vi "TCP.IP Server for Ripple Detection - Experiment 6.vi"() -> ()   [LabVIEW 2021]
doc: "Demonstrates how to set up a basic TCP connection, send data to the specified port once a connection has been established, and terminate the connection once the data has been sent. This VI is designed to stop if the TCP connection is terminated. The data sent in this example is an array of random numbers."
panel:
  in  "Number of row to read \nat a time":i32=10000
  in  "File Path":path
  out "Iteration terminal":i32
  in  "Stop 2":bool
  in  "Client Closed":string="The client VI closed the connection."
  in  "Stop":bool
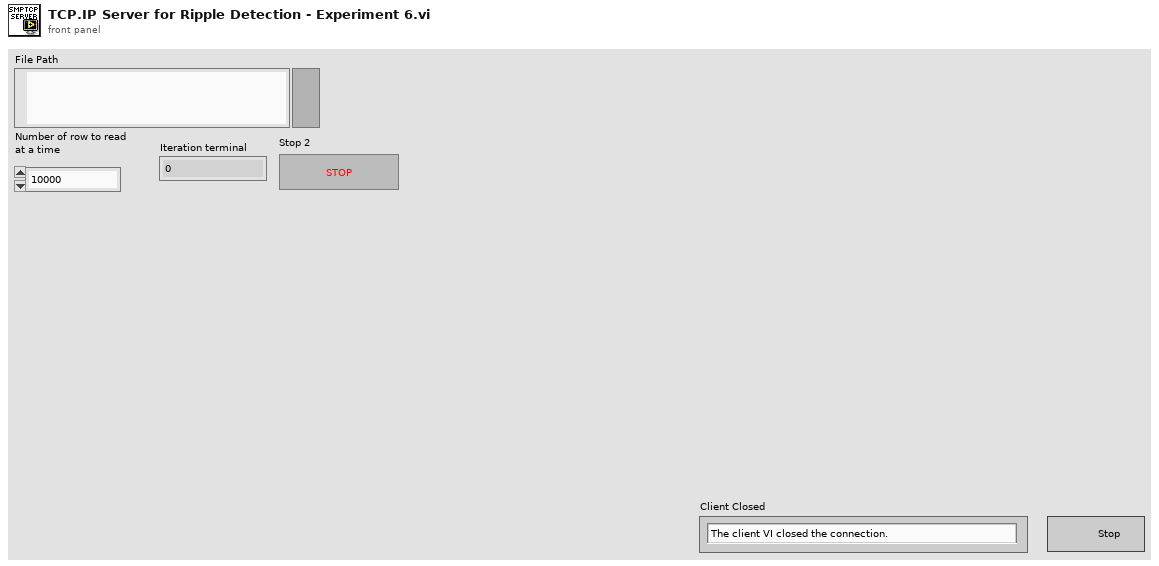
[diagram p1: front panel]
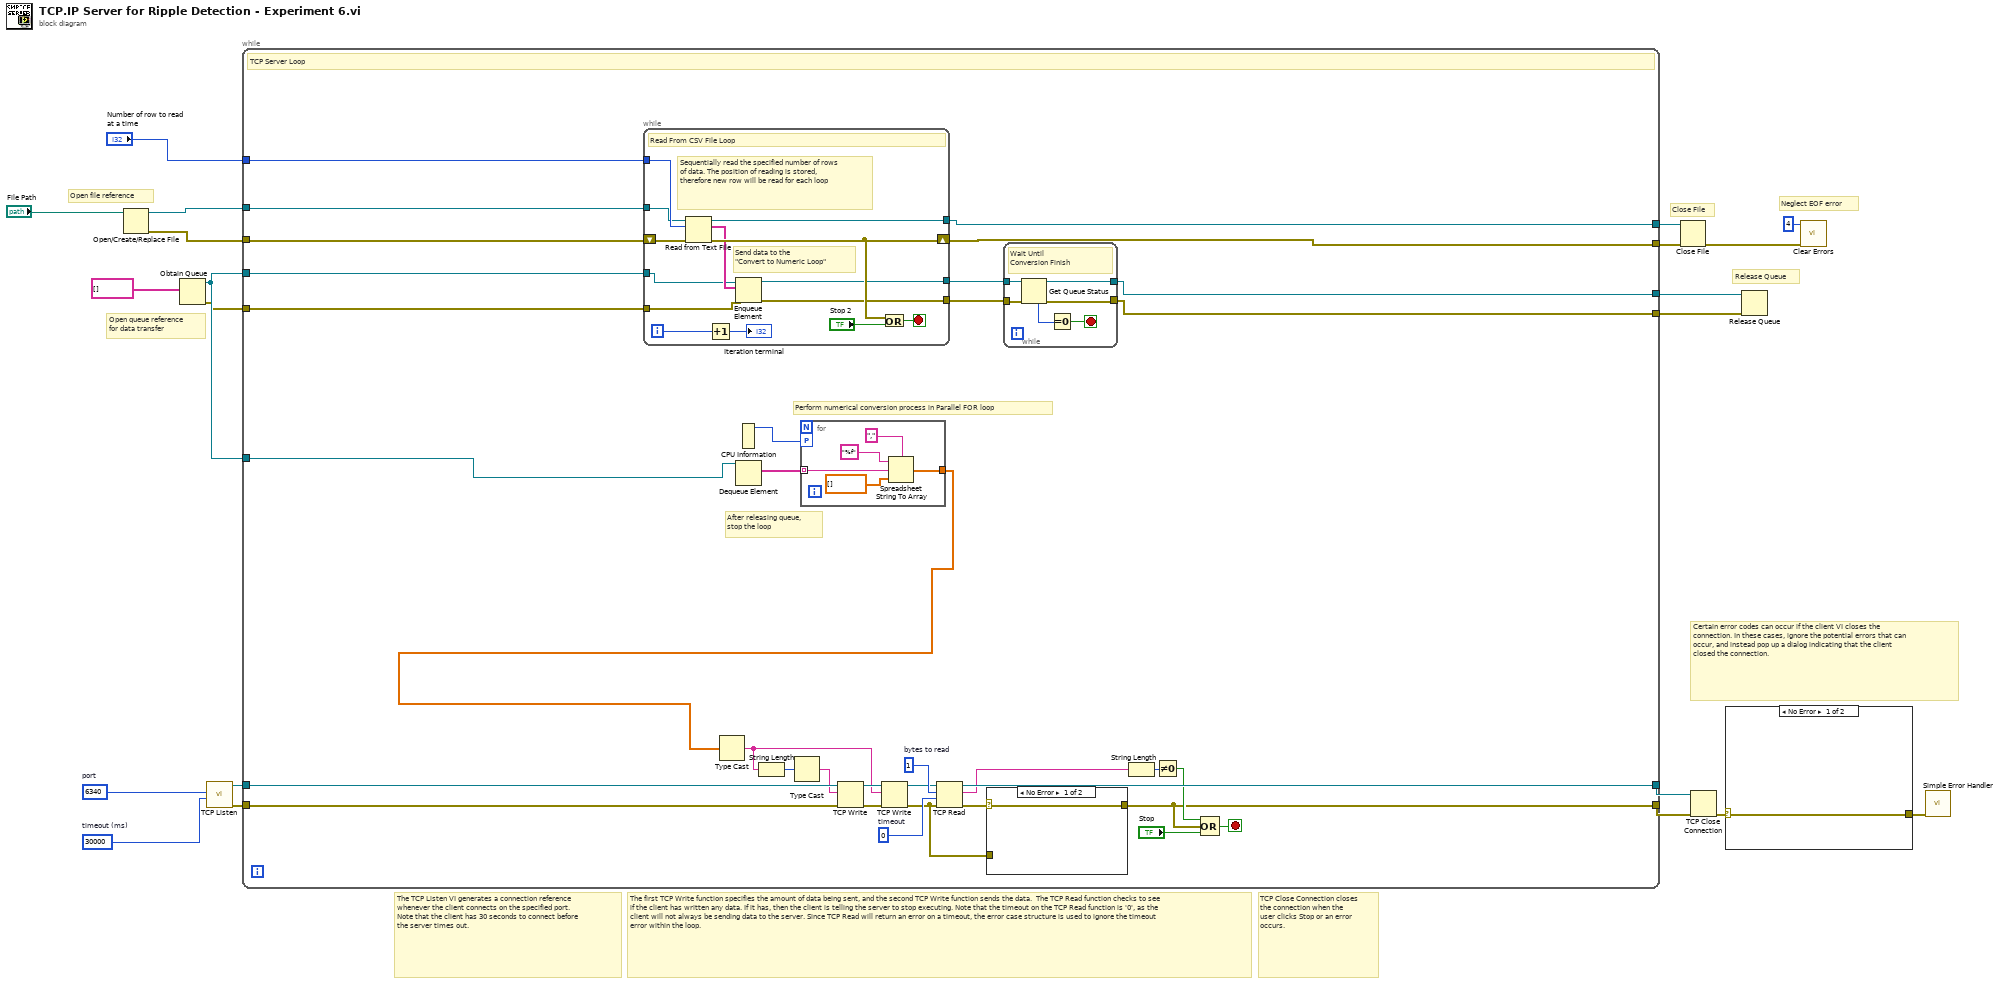
[diagram p0: block diagram]
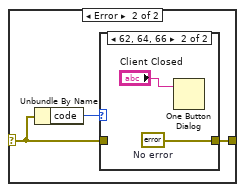
[diagram p2: hidden frame]
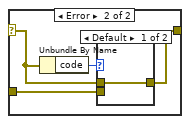
[diagram p4: hidden frame]
diagram:
  w14 = u16 6340  # port
  w15 = 30000  # timeout (ms)
  # "Open queue reference\nfor data transfer"
  # "Release Queue"
  # "Neglect EOF error"
  # "Close File"
  # "Open file reference"
  # "TCP Close Connection closes the connection when the user clicks Stop or an error occurs."
  # "The TCP Listen VI generates a connection reference whenever the client connects on the specified port. Note that the client has 30 seconds to connect before the server times out."
  # "Certain error codes can occur if the client VI closes the connection. In these cases, ignore the potential errors that can occur, and instead pop up a dialog indicating that the client closed the connection."
  # "The first TCP Write function specifies the amount of data being sent, and the second TCP Write function sends the data.  The TCP Read function checks to see if the client has written any data. If it has, then the client is telling the server to stop executing. Note that the timeout on the TCP Read function is '0', as the client will not always be sending data to the server. Since TCP Read will return an error on a timeout, the error case structure is used to ignore the timeout error within the loop."
  n1 = Open/Create/Replace File(file path (use dialog)="File Path") -> (refnum out=w11:refnum<file>, error out=w12:errorcluster)  [unwired: 5 in, 1 out]
  n2 = Obtain Queue(element data type=string[] [] ("形式文字列")) -> (queue out=w3:refnum<queue>, error out=w2:errorcluster)  [unwired: 4 in, 1 out]
  n3 = call <vilib>:"TCP Listen.vi"("timeout ms (wait forever: -1)"=w15, "port"=w14) -> ("error out"=w16:errorcluster, "connection ID"=w17:refnum<k5>)  [unwired: 5 in, 3 out]
  n4 = while {
    tunnel: [w38] -> w20
    tunnel: [w44] -> w21
    tunnel: w17 -> [w55]
    tunnel: w16 -> [w48]
    tunnel: w11 -> [w34]
    tunnel: w12 -> [w33]
    tunnel: [w32] -> w9
    tunnel: [w31] -> w8
    tunnel: [w30] -> w6
    tunnel: [w29] -> w5
    tunnel: w3 -> [w23]
    tunnel: w3 -> [w28]
    tunnel: w2 -> [w27]
    tunnel: "Number of row to read \nat a time" -> [w26]
    stop <- w49 stop-if-true
    w43 = 0  # timeout
    w46 = 1  # bytes to read
    # "After releasing queue,\nstop the loop"
    # "Perform numerical conversion process in Parallel FOR loop"
    # "TCP Server Loop"
    n5 = while {
      tunnel: [w79] -> w31
      shift-right: [w74] -> w32
      shift-left: w33 -> [w80]
      tunnel: w26 -> [w75]
      tunnel: [w72] -> w35
      tunnel: [w71] -> w36
      tunnel: w34 -> [w69]
      tunnel: w28 -> [w68]
      tunnel: w27 -> [w67]
      i -> [w77]
      stop <- w78 stop-if-true
      # "Send data to the \n\"Convert to Numeric Loop\""
      # "Sequentially read the specified number of rows of data. The position of reading is stored, therefore new row will be read for each loop"
      # "Read From CSV File Loop"
      n6 = Read from Text File(file (use dialog)=w69, count=w75, error in=w80) -> (refnum out=w79:refnum<file>, text=w73:string[], error out=w74:errorcluster)  [unwired: 1 in, 1 out]
      n7 = Increment(x=w77) -> (x+1=→"Iteration terminal":i32)
      n8 = Enqueue Element(queue=w68, element=w73, error in (no error)=w67) -> (queue out=w72:refnum<queue>, error out=w71:errorcluster)  [unwired: 1 in, 1 out]
      n9 = Or(x=w74, y="Stop 2") -> (x .or. y?=w78:bool)
    }
    n10 = CPU Information() -> (4:w25:i32)  [unwired: 3 out]
    n11 = Dequeue Element(queue=w23) -> (element=w24:string[])  [unwired: 2 in, 3 out]
    n12 = for "Forループ" {
      tunnel: w24 -> [w57] mode=indexing
      tunnel: [w58] -> w22
      workers-P: w25 -> [_]
      n13 = Spreadsheet String To Array(delimiter (Tab)="," ("デリミタ（タブ）"), format string="%f" ("形式文字列"), spreadsheet string=w57, array type (2D Dbl)=dbl[] []) -> (array=w58:dbl[])
    }
    n14 = Type Cast(x=w22) -> (*(type *) &x=w50:string)  [unwired: 1 out]
    n15 = String Length(string=w50) -> (length=w52:i32)
    n16 = Type Cast(x=w52) -> (*(type *) &x=w51:string)  [unwired: 1 out]
    n17 = TCP Write(connection ID=w55, data in=w51, error in (no error)=w48) -> (connection ID out=w54:refnum<k5>, error out=w53:errorcluster)  [unwired: 2 out]
    n18 = TCP Write(connection ID=w54, data in=w50, error in (no error)=w53) -> (connection ID out=w45:refnum<k5>, error out=w37:errorcluster)  [unwired: 2 out]
    n19 = TCP Read(connection ID=w45, bytes to read=w46, error in (no error)=w37, 9:w43) -> (connection ID out=w44:refnum<k5>, data out=w41:string, error out=w39:errorcluster)  [unwired: 1 out]
    n20 = case shown="No Error" w39 {
      selector: w39 -> [w81 w84]
      tunnel: [w81 w82] -> w38
      tunnel: w37 -> [_ w83]
      frame No Error {
      }
      frame Error {
        n21 = Unbundle By Name(w84) -> ("code"=w85:i32)
        n22 = case shown="Default" w85 {
          tunnel: w84 -> [w86 _]
          tunnel: w83 -> [_ w87]
          tunnel: [w86 w87] -> w82
          frame Default {
          }
          frame 56 {
          }
        }
      }
    }
    n23 = while {
      tunnel: w35 -> [w66]
      tunnel: w36 -> [w65]
      tunnel: [w62] -> w30
      tunnel: [w61] -> w29
      stop <- w63 stop-if-true
      # "Wait Until \nConversion Finish"
      n24 = Get Queue Status(queue=w66, error in (no error)=w65) -> (queue out=w62:refnum<queue>, error out=w61:errorcluster, # elements in queue=w64:i32)  [unwired: 1 in, 5 out]
      n25 = Equal To 0?(x=w64) -> (x = 0?=w63:bool)
    }
    n26 = String Length(string=w41) -> (length=w42:i32)
    n27 = Not Equal To 0?(x=w42) -> (x != 0?=w40:bool)
    n28 = Compound Arithmetic op=OR(w40, w38, "Stop") -> (w49:bool)
  }
  n29 = Close File(refnum=w8, error in=w9) -> (error out=w10:errorcluster)  [unwired: 1 out]
  n30 = TCP Close Connection(connection ID=w21, error in (no error)=w20) -> (error out=w19:errorcluster)  [unwired: 2 out]
  n31 = case shown="No Error" w19 {
    selector: w19 -> [w88 w90]
    tunnel: [w88 w89] -> w18
    frame No Error {
    }
    frame Error {
      n32 = Unbundle By Name(w90) -> ("code"=w91:i32)
      n33 = case shown="62, 64, 66" w91 {
        tunnel: w90 -> [w92 _]
        tunnel: [w92 w94] -> w89
        frame Default {
        }
        frame 62, 64, 66 {
          w94 = errorcluster {"status"=FALSE, "code"=0, "source"=""}  # No error
          n34 = One Button Dialog(message="Client Closed") -> ()  [unwired: 1 in, 1 out]
        }
      }
    }
  }
  n35 = Release Queue(queue=w6, error in (no error)=w5) -> ()  [unwired: 1 in, 3 out]
  n36 = call <vilib>:"Clear Errors.vi"("error in (no error)"=w10, "specific error code to clear (0: all)"=4) -> ()  [unwired: 4 in, 2 out]
  n37 = call <vilib>:"Simple Error Handler.vi"("error in (no error)"=w18) -> ()  [unwired: 1 in, 8 out]
